vi "Move XYZ.vi"(0 "PID Gains In":T1={"X PID"={"proportional gain (Kc)"=0.03, "integral time (Ti, min)"=0.0, "derivative time (Td, min)"=0.0}, "Y PID"={"proportional gain (Kc)"=0.03, "integral time (Ti, min)"=0.0, "derivative time (Td, min)"=0.0}, "Z PID"={"proportional gain (Kc)"=0.035, "integral time (Ti, min)"=0.0, "derivative time (Td, min)"=0.0}} {"Z PID"."derivative time (Td, min)" format="%.3f"; "Z PID"."integral time (Ti, min)" format="%.3f"; "Z PID"."proportional gain (Kc)" format="%.3f"; "Y PID"."derivative time (Td, min)" format="%.3f"; "Y PID"."integral time (Ti, min)" format="%.3f"; "Y PID"."proportional gain (Kc)" format="%.3f"; "X PID"."derivative time (Td, min)" format="%.3f"; "X PID"."integral time (Ti, min)" format="%.3f"; "X PID"."proportional gain (Kc)" format="%.3f"}, 5 "Y Target":dbl, 6 "X Target":dbl, 10 "Max Time":dbl=90.0, 11 "Gyro Target":dbl=-180.0, 12 "Movement":dbl=3.0, 14 "X Output Range":cluster{"output high":dbl, "output low":dbl}={"output high"=0.8, "output low"=-0.8}, 15 "X Stop Threshold":dbl=5.0, 16 "Y Output Range":cluster{"output high":dbl, "output low":dbl}={"output high"=0.8, "output low"=-0.8}, 17 "Y Stop Threshold":dbl=5.0, 18 "Z Output Range":cluster{"output high":dbl, "output low":dbl}={"output high"=0.8, "output low"=-0.8}, 19 "Z  Stop Threshold":dbl=8.0) -> ()   [LabVIEW 2018]
uses:
  Robot Global Data.vi
  SubSystems/Drive Train/Drive Train Global.vi
  SubSystems/Hatch Panel Intake/Hatch Panel Intake Global.vi
  SubSystems/Lift/Lift Global.vi
  <vilib>/addons/control/pid/pid.llb/PID (DBL).vi
  <vilib>/addons/control/pid/NI_PID_pid.lvlib
panel:
  in  "Minimum Time":u32=500
  in  "Settle Time":u32=2000
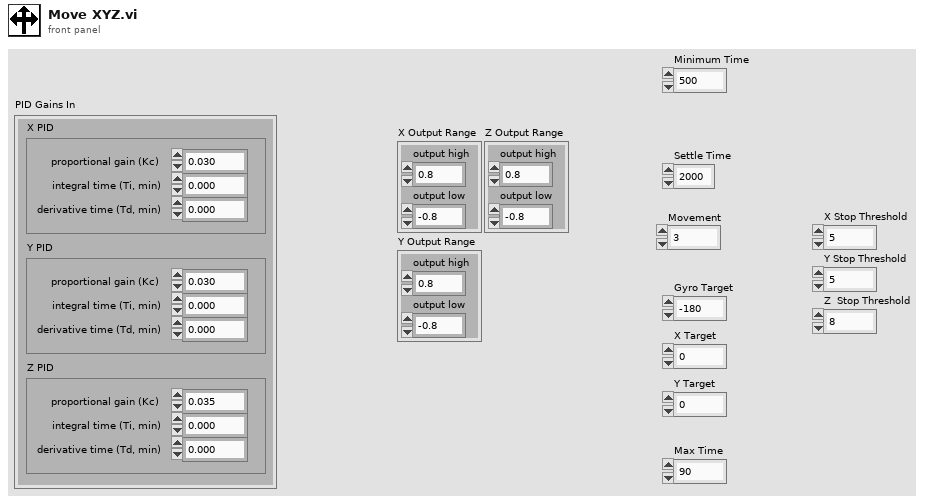
[diagram p1: front panel]
types:
  T1 = cluster{"X PID":cluster{"proportional gain (Kc)":dbl, "integral time (Ti, min)":dbl, "derivative time (Td, min)":dbl}, "Y PID":cluster{"proportional gain (Kc)":dbl, "integral time (Ti, min)":dbl, "derivative time (Td, min)":dbl}, "Z PID":cluster{"proportional gain (Kc)":dbl, "integral time (Ti, min)":dbl, "derivative time (Td, min)":dbl}}
  T2 = cluster{"proportional gain (Kc)":dbl, "integral time (Ti, min)":dbl, "derivative time (Td, min)":dbl}
  T3 = cluster{"Rollover":dbl, "Yaw":dbl, "Cont Yaw":dbl}
  T4 = cluster{"offsetAngle H":dbl, "offsetAngle V":dbl, "area":dbl, "skew":dbl, "validTarget":dbl, "latency":dbl}
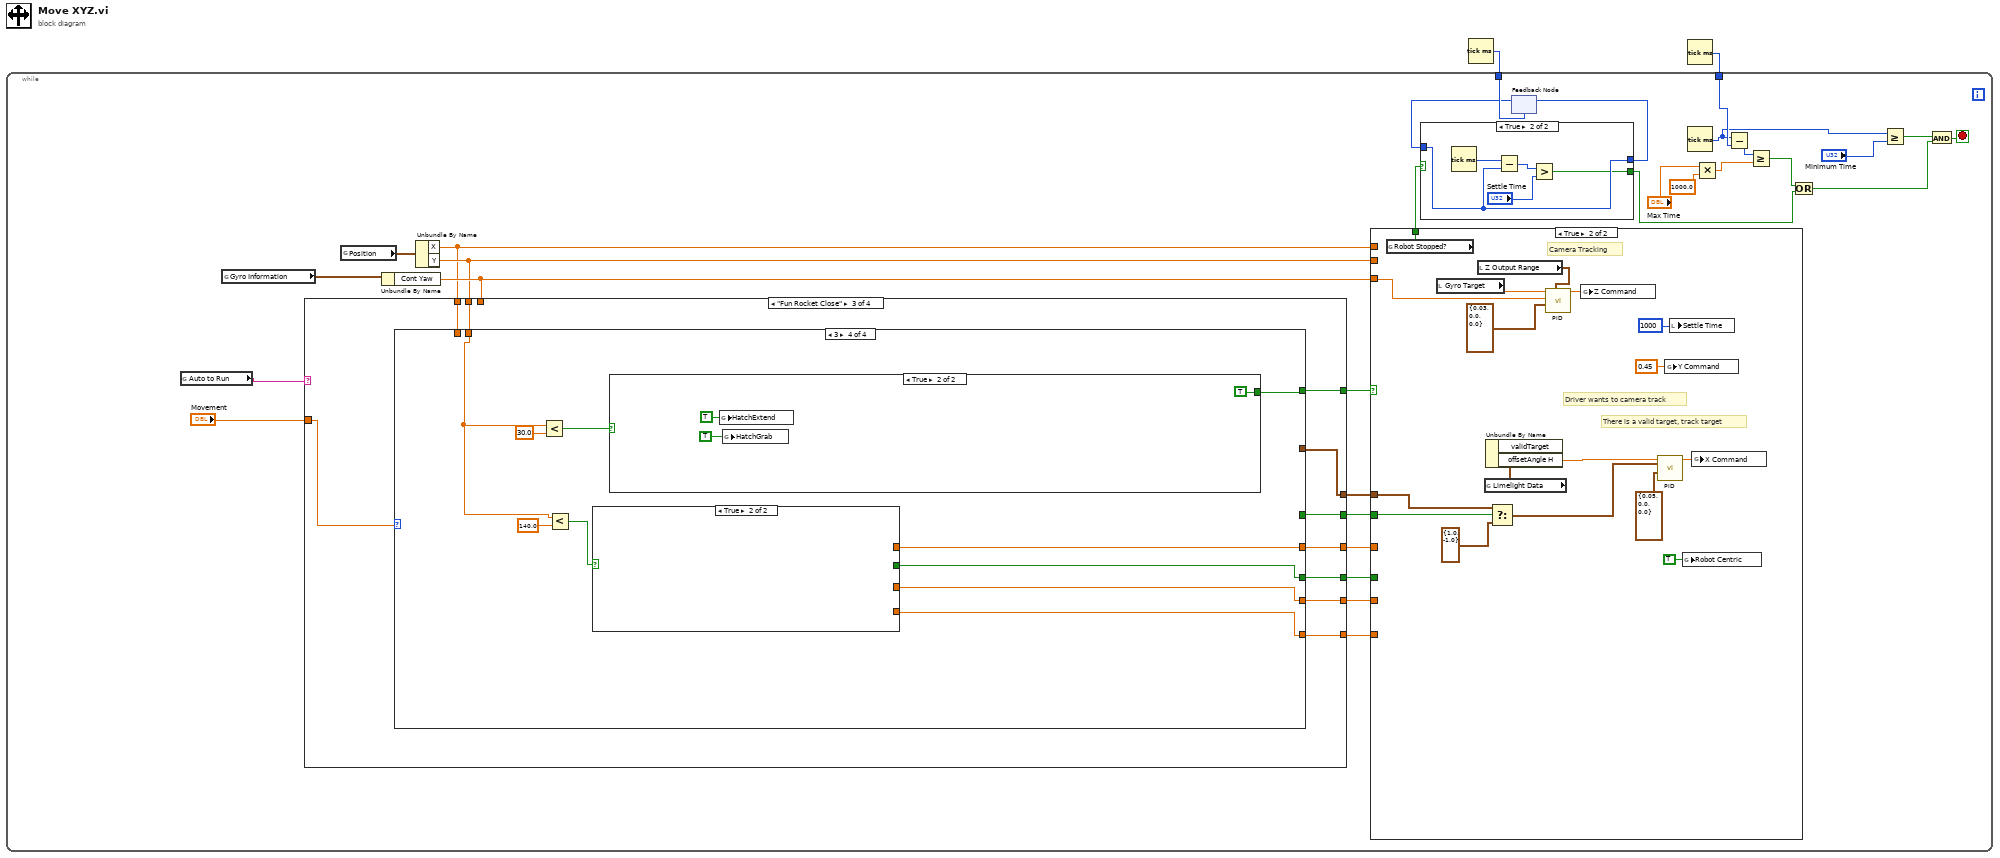
[diagram p0: block diagram]
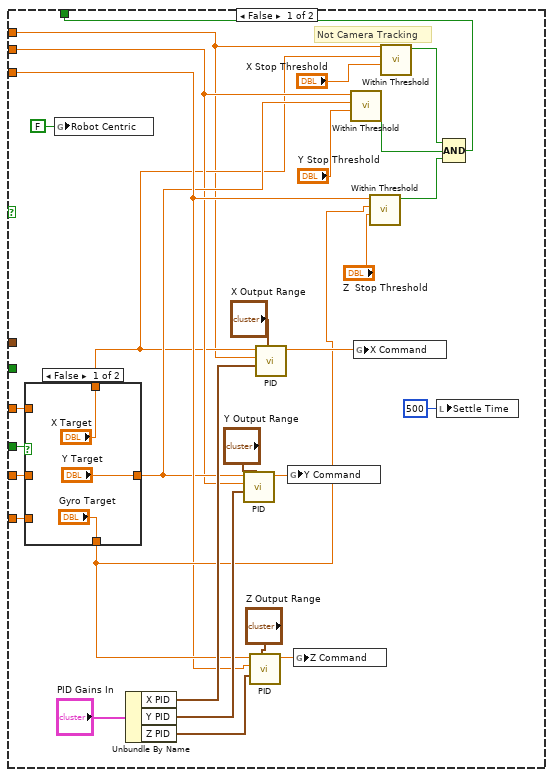
[diagram p2: hidden frame]
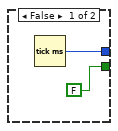
[diagram p4: hidden frame]
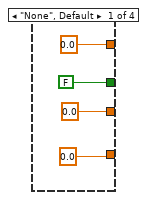
[diagram p5: hidden frame]
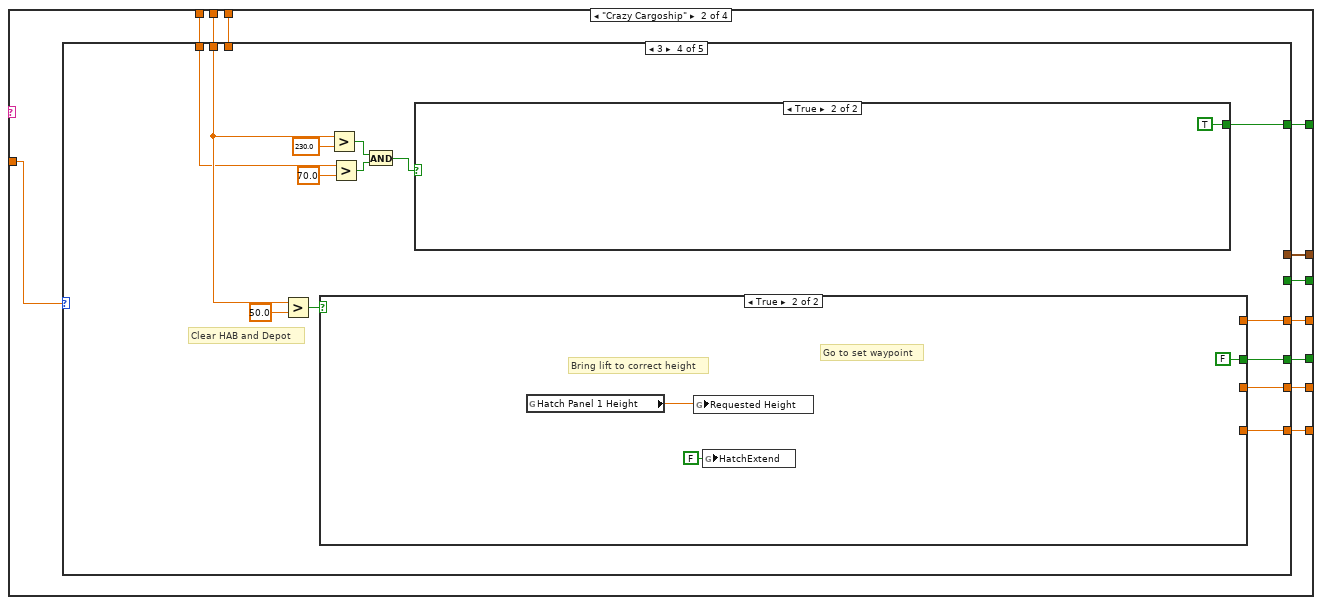
[diagram p6: hidden frame]
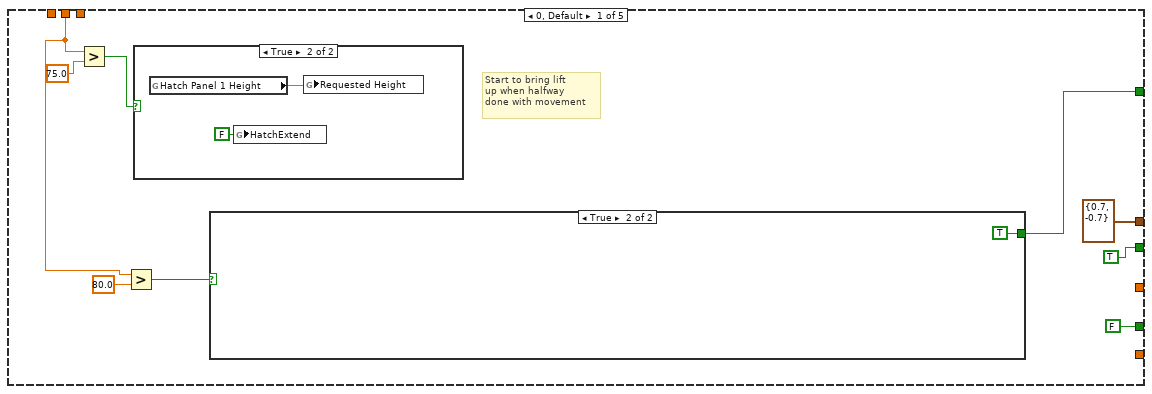
[diagram p7: hidden frame]
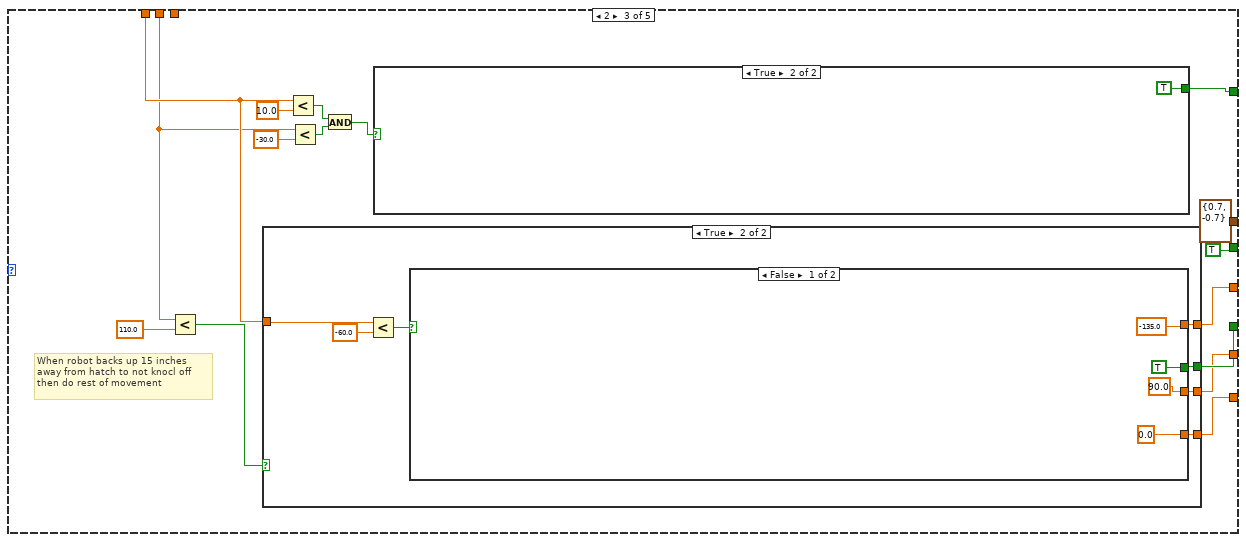
[diagram p11: hidden frame]
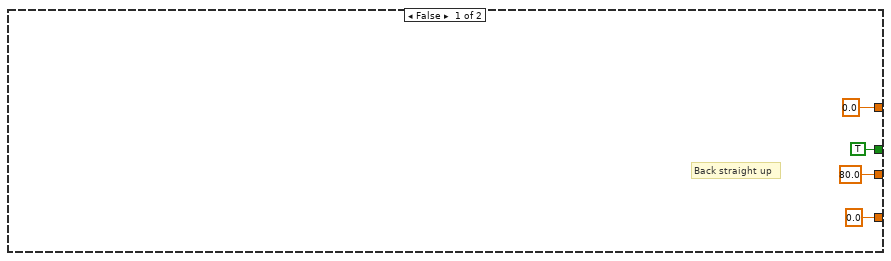
[diagram p13: hidden frame]
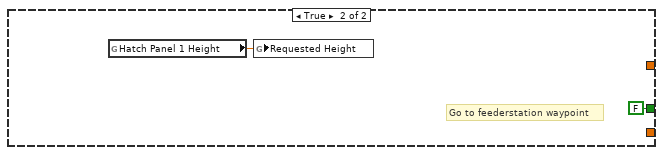
[diagram p14: hidden frame]
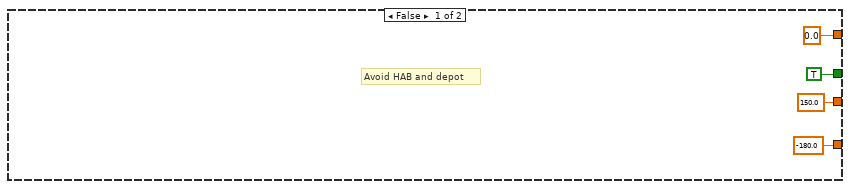
[diagram p16: hidden frame]
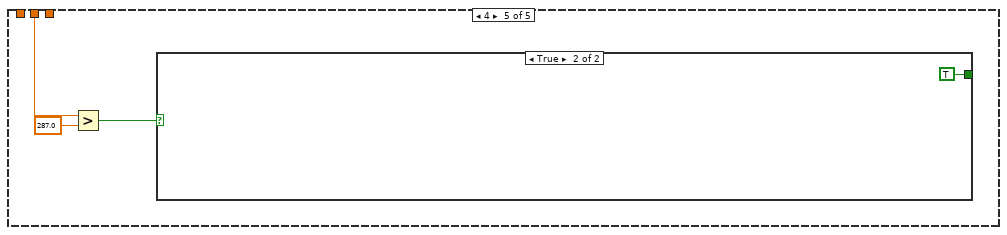
[diagram p17: hidden frame]
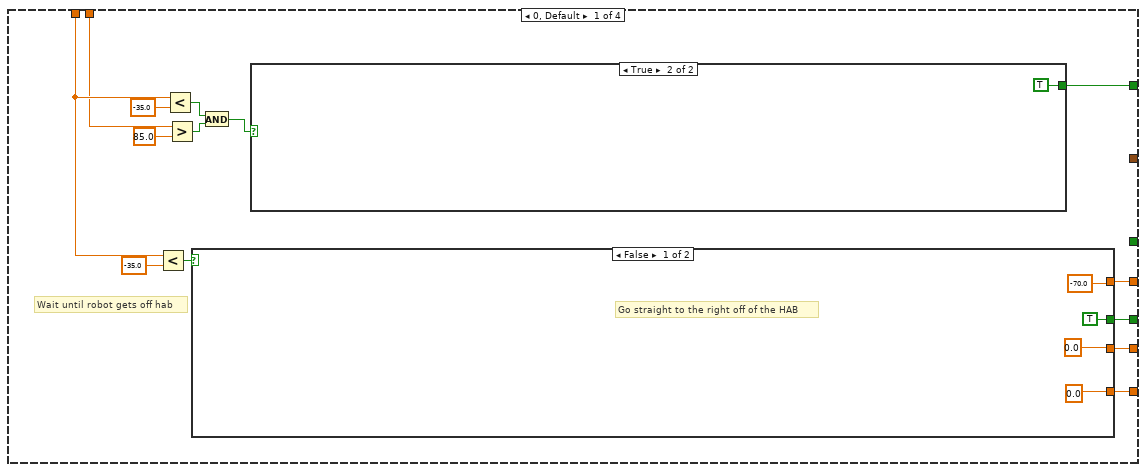
[diagram p19: hidden frame]
diagram:
  n1 = Tick Count (ms)() -> (millisecond timer value=w2:u32)
  n2 = Tick Count (ms)() -> (millisecond timer value=w1:u32)
  n3 = while {
    tunnel: w2 -> [w26]
    tunnel: w1 -> [w11]
    stop <- w10 stop-if-true
    n4 = global read "Robot Global Data.vi" "Auto to Run"() -> (w23:string)
    n5 = global read "Drive Train Global.vi" "Gyro Information"() -> (w20:T3)
    n6 = global read "Drive Train Global.vi" "Position"() -> (w22:cluster{"X":dbl, "Y":dbl})
    n7 = Unbundle By Name(w20) -> ("Cont Yaw"=w18:dbl)
    n8 = Unbundle By Name(w22) -> ("X"=w16:dbl, "Y"=w17:dbl)
    n9 = case shown="\"Fun Rocket Close\"" w23 {
      tunnel: [0.0 w101 w184 w266] -> w32
      tunnel: [0.0 w100 w183 w265] -> w31
      tunnel: [0.0 w99 w182 w264] -> w30
      tunnel: w17 -> [_ w105 w187 w269]
      tunnel: [FALSE w104 w185 w267] -> w29
      tunnel: w16 -> [_ w102 w186 w268]
      tunnel: "Movement" -> [_ w106 w188 w270]
      tunnel: w18 -> [_ w103 _ w262]
      tunnel: [_ w98 w181 w263] -> w5
      tunnel: [_ w96 w179 _] -> w4
      tunnel: [_ w97 w180 _] -> w3
      frame "None", Default {
      }
      frame "Crazy Cargoship" {
        n10 = case shown="3" w106 {
          tunnel: w105 -> [w109 _ w121 w154 w175]
          tunnel: [FALSE _ w132 w166 _] -> w104
          tunnel: w103 -> [_ _ _ _ _]
          tunnel: w102 -> [_ _ w122 w153 _]
          tunnel: [_ _ w131 w163 _] -> w101
          tunnel: [_ _ w130 w162 _] -> w100
          tunnel: [_ _ w129 w161 _] -> w99
          tunnel: [w111 _ w123 w155 _] -> w98
          tunnel: [TRUE ("Robot Centric") _ TRUE ("Robot Centric") _ _] -> w97
          tunnel: [cluster{"output high":dbl, "output low":dbl} {"output high"=0.7, "output low"=-0.7} ("output range") _ cluster{"output high":dbl, "output low":dbl} {"output high"=0.7, "output low"=-0.7} ("output range") _ _] -> w96
          frame 0, Default {
            # "Start to bring lift\nup when halfway\ndone with movement"
            n11 = Greater?(x=w109, y=75.0) -> (0:w114:bool)
            n12 = Greater?(x=w109, y=80.0) -> (0:w110:bool)
            n13 = case shown="True" w114 {
              frame False {
              }
              frame True {
                n14 = global read "Lift Global.vi" "Hatch Panel 1 Height"() -> (w118:dbl)
                n15 = global write "Hatch Panel Intake Global.vi" "HatchExtend"(FALSE ("HatchGrab")) -> ()
                n16 = global write "Lift Global.vi" "Requested Height"(w118) -> ()
              }
            }
            n17 = case shown="True" w110 {
              tunnel: [_ TRUE] -> w111
              frame False {
              }
              frame True {
              }
            }
          }
          frame 1 {
          }
          frame 2 {
            # "When robot backs up 15 inches\naway from hatch to not knocl off\nthen do rest of movement"
            n18 = Less?(x=w121, y=110.0) -> (x < y?=w134:bool)
            n19 = case shown="True" w134 {
              tunnel: [TRUE w146] -> w132
              tunnel: [0.0 w142] -> w131
              tunnel: [80.0 w141] -> w130
              tunnel: [0.0 w140] -> w129
              tunnel: w122 -> [_ w143]
              frame False {
                # "Back straight up"
              }
              frame True {
                n20 = Less?(x=w143, y=-60.0) -> (x < y?=w144:bool)
                n21 = case shown="False" w144 {
                  tunnel: [TRUE FALSE] -> w146
                  tunnel: [-135.0 _] -> w142
                  tunnel: [90.0 _] -> w141
                  tunnel: [0.0 _] -> w140
                  frame False {
                  }
                  frame True {
                    # "Go to feederstation waypoint"
                    n22 = global read "Lift Global.vi" "Hatch Panel 1 Height"() -> (w151:dbl)
                    n23 = global write "Lift Global.vi" "Requested Height"(w151) -> ()
                  }
                }
              }
            }
            n24 = Less?(x=w122, y=10.0) -> (x < y?=w126:bool)
            n25 = Less?(x=w121, y=-30.0) -> (x < y?=w125:bool)
            n26 = And(x=w126, y=w125) -> (x .and. y?=w124:bool)
            n27 = case shown="True" w124 {
              tunnel: [_ TRUE] -> w123
              frame False {
              }
              frame True {
              }
            }
          }
          frame 3 {
            # "Clear HAB and Depot"
            n28 = Greater?(x=w154, y=50.0) -> (0:w165:bool)
            n29 = case shown="True" w165 {
              tunnel: [TRUE FALSE] -> w166
              tunnel: [0.0 _] -> w163
              tunnel: [150.0 _] -> w162
              tunnel: [-180.0 _] -> w161
              frame False {
                # "Avoid HAB and depot"
              }
              frame True {
                # "Bring lift to correct height"
                # "Go to set waypoint"
                n30 = global read "Lift Global.vi" "Hatch Panel 1 Height"() -> (w173:dbl)
                n31 = global write "Lift Global.vi" "Requested Height"(w173) -> ()
                n32 = global write "Hatch Panel Intake Global.vi" "HatchExtend"(FALSE ("HatchGrab")) -> ()
              }
            }
            n33 = Greater?(x=w154, y=230.0) -> (0:w158:bool)
            n34 = Greater?(x=w153, y=70.0) -> (0:w157:bool)
            n35 = And(x=w158, y=w157) -> (x .and. y?=w156:bool)
            n36 = case shown="True" w156 {
              tunnel: [_ TRUE] -> w155
              frame False {
              }
              frame True {
              }
            }
          }
          frame 4 {
            n37 = Greater?(x=w175, y=287.0) -> (0:w176:bool)
            n38 = case shown="True" w176 {
              tunnel: [_ TRUE] -> _
              frame False {
              }
              frame True {
              }
            }
          }
        }
      }
      frame "Fun Rocket Close" {
        n39 = case shown="3" w188 {
          tunnel: w187 -> [w195 w210 w229 w250]
          tunnel: w186 -> [w196 w215 _ _]
          tunnel: [w200 _ w227 w245] -> w185
          tunnel: [w199 _ w228 w248] -> w184
          tunnel: [w198 _ w226 w247] -> w183
          tunnel: [w197 _ w225 w246] -> w182
          tunnel: [w189 w216 w235 w253] -> w181
          tunnel: [_ _ w233 _] -> w180
          tunnel: [_ _ w232 _] -> w179
          frame 0, Default {
            # "Wait until robot gets off hab"
            n40 = Less?(x=w196, y=-35.0) -> (x < y?=w202:bool)
            n41 = Less?(x=w196, y=-35.0) -> (x < y?=w192:bool)
            n42 = Greater?(x=w195, y=85.0) -> (0:w191:bool)
            n43 = case shown="False" w202 {
              tunnel: [TRUE FALSE] -> w200
              tunnel: [-70.0 _] -> w199
              tunnel: [0.0 _] -> w198
              tunnel: [0.0 _] -> w197
              frame False {
                # "Go straight to the right off of the HAB"
              }
              frame True {
                # "Bring the lift up to the correct level because its slow"
                # "Robot off of HAB, go to the rocket"
                n44 = global read "Lift Global.vi" "Hatch Panel 2 Height"() -> (w208:dbl)
                n45 = global write "Lift Global.vi" "Requested Height"(w208) -> ()
              }
            }
            n46 = And(x=w192, y=w191) -> (x .and. y?=w190:bool)
            n47 = case shown="True" w190 {
              tunnel: [_ TRUE] -> w189
              frame False {
              }
              frame True {
              }
            }
          }
          frame 1 {
            n48 = Less?(x=w210, y=-17.0) -> (x < y?=w219:bool)
            n49 = Less?(x=w215, y=-90.0) -> (x < y?=w218:bool)
            n50 = Less?(x=w210, y=0.0) -> (x < y?=w213:bool)
            n51 = Less?(x=w210, y=-5.0) -> (x < y?=w212:bool)
            n52 = And(x=w219, y=w218) -> (x .and. y?=w217:bool)
            n53 = case shown="True" w213 {
              frame False {
              }
              frame True {
                n54 = global write "Hatch Panel Intake Global.vi" "HatchExtend"(TRUE ("HatchExtend")) -> ()
              }
            }
            n55 = case shown="True" w212 {
              frame False {
              }
              frame True {
                n56 = global write "Hatch Panel Intake Global.vi" "HatchGrab"(TRUE ("HatchExtend")) -> ()
              }
            }
            n57 = case shown="True" w217 {
              tunnel: [_ TRUE] -> w216
              frame False {
              }
              frame True {
              }
            }
          }
          frame 2 {
            # "back up then turn"
            n58 = Greater?(x=w229, y=150.0) -> (0:w234:bool)
            n59 = Greater?(x=w229, y=40.0) -> (0:w230:bool)
            n60 = case shown="True" w234 {
              tunnel: [_ TRUE] -> w235
              tunnel: [_ TRUE] -> w233
              tunnel: [_ cluster{"output high":dbl, "output low":dbl} {"output high"=0.6, "output low"=-0.6} ("output range")] -> w232
              frame False {
              }
              frame True {
              }
            }
            n61 = case shown="False" w230 {
              tunnel: [0.0 _] -> w228
              tunnel: [TRUE FALSE] -> w227
              tunnel: [200.0 _] -> w226
              tunnel: [-180.0 _] -> w225
              frame False {
              }
              frame True {
              }
            }
          }
          frame 3 {
            n62 = Less?(x=w250, y=30.0) -> (x < y?=w252:bool)
            n63 = Less?(x=w250, y=140.0) -> (x < y?=w249:bool)
            n64 = case shown="True" w249 {
              tunnel: [0.0 _] -> w248
              tunnel: [100.0 _] -> w247
              tunnel: [-30.0 _] -> w246
              tunnel: [TRUE _] -> w245
              frame False {
              }
              frame True {
              }
            }
            n65 = case shown="True" w252 {
              tunnel: [_ TRUE] -> w253
              frame False {
              }
              frame True {
                n66 = global write "Hatch Panel Intake Global.vi" "HatchExtend"(TRUE ("HatchExtend")) -> ()
                n67 = global write "Hatch Panel Intake Global.vi" "HatchGrab"(TRUE ("HatchExtend")) -> ()
              }
            }
          }
        }
      }
      frame "Fun Rocket Far" {
        n68 = case shown="2" w270 {
          tunnel: w269 -> [w273 w307 w326 w342]
          tunnel: w268 -> [w272 w305 _ _]
          tunnel: [w277 w303 w331 w337] -> w267
          tunnel: [w276 w304 w330 w340] -> w266
          tunnel: [w275 w302 w329 w339] -> w265
          tunnel: [w274 w301 w328 w338] -> w264
          tunnel: [w271 w310 _ w345] -> w263
          tunnel: w262 -> [_ _ _ _]
          frame 0, Default {
            # "Wait until robot gets off hab"
            n69 = Greater?(x=w273, y=160.0) -> (0:w279:bool)
            n70 = case shown="True" w279 {
              tunnel: [TRUE w292] -> w277
              tunnel: [-10.0 w290] -> w276
              tunnel: [170.0 w289] -> w275
              tunnel: [0.0 w288] -> w274
              tunnel: w272 -> [_ w285]
              tunnel: [_ w284] -> w271
              frame False {
              }
              frame True {
                # "Bring the lift up to the correct level because its slow"
                n71 = global read "Lift Global.vi" "Hatch Panel 2 Height"() -> (w291:dbl)
                n72 = global write "Lift Global.vi" "Requested Height"(w291) -> ()
                n73 = Less?(x=w285, y=-60.0) -> (x < y?=w286:bool)
                n74 = case shown="False" w286 {
                  tunnel: [TRUE FALSE] -> w292
                  tunnel: [-100.0 ("y") _] -> w290
                  tunnel: [195.0 ("y") _] -> w289
                  tunnel: [-150.0 ("y") _] -> w288
                  tunnel: [_ TRUE] -> w284
                  frame False {
                  }
                  frame True {
                  }
                }
              }
            }
          }
          frame 1 {
            n75 = Less?(x=w307, y=-30.0) -> (x < y?=w313:bool)
            n76 = Greater?(x=w305, y=65.0) -> (0:w312:bool)
            n77 = Less?(x=w307, y=0.0) -> (x < y?=w308:bool)
            n78 = And(x=w313, y=w312) -> (x .and. y?=w311:bool)
            n79 = case shown="True" w308 {
              frame False {
              }
              frame True {
                n80 = global write "Hatch Panel Intake Global.vi" "HatchExtend"(TRUE ("HatchExtend")) -> ()
                n81 = global write "Hatch Panel Intake Global.vi" "HatchGrab"(TRUE ("HatchExtend")) -> ()
              }
            }
            n82 = Greater?(x=w305, y=-40.0) -> (0:w299:bool)
            n83 = case shown="False" w311 {
              tunnel: [FALSE TRUE] -> w310
              frame False {
              }
              frame True {
              }
            }
            n84 = call "Flip Flop.vi"("Line 1"=w299) -> ("Switch"=w300:bool)  [unwired: 10 in]
            n85 = case shown="True" w300 {
              tunnel: [_ -30.0 ("y")] -> w304
              tunnel: [FALSE TRUE] -> w303
              tunnel: [_ 190.0 ("y")] -> w302
              tunnel: [_ -150.0 ("y")] -> w301
              frame False {
              }
              frame True {
              }
            }
          }
          frame 2 {
            n86 = Less?(x=w326, y=30.0) -> (x < y?=w327:bool)
            n87 = case shown="False" w327 {
              tunnel: [TRUE FALSE] -> w331
              tunnel: [-30.0 _] -> w330
              tunnel: [100.0 _] -> w329
              tunnel: [-180.0 _] -> w328
              frame False {
              }
              frame True {
              }
            }
          }
          frame 3 {
            n88 = Less?(x=w342, y=30.0) -> (x < y?=w344:bool)
            n89 = Less?(x=w342, y=140.0) -> (x < y?=w341:bool)
            n90 = case shown="False" w341 {
              tunnel: [0.0 _] -> w340
              tunnel: [100.0 _] -> w339
              tunnel: [-30.0 _] -> w338
              tunnel: [TRUE _] -> w337
              frame False {
              }
              frame True {
              }
            }
            n91 = case shown="True" w344 {
              tunnel: [_ TRUE] -> w345
              frame False {
              }
              frame True {
              }
            }
          }
        }
      }
    }
    n92 = case shown="True" w5 {
      tunnel: w32 -> [w54 _]
      tunnel: w31 -> [w53 _]
      tunnel: w30 -> [w52 _]
      tunnel: w29 -> [w51 _]
      tunnel: [w35 w68] -> w19
      tunnel: w18 -> [w45 w75]
      tunnel: w17 -> [w41 _]
      tunnel: w16 -> [w37 _]
      tunnel: w4 -> [_ w71]
      tunnel: w3 -> [_ w70]
      frame False {
        # "Not Camera Tracking"
        n93 = case shown="False" w51 {
          tunnel: ["X Target" w67] -> w38
          tunnel: ["Y Target" w66] -> w42
          tunnel: ["Gyro Target" w65] -> w46
          tunnel: w54 -> [_ w67]
          tunnel: w53 -> [_ w66]
          tunnel: w52 -> [_ w65]
          frame False {
          }
          frame True {
          }
        }
        n94 = global write "Drive Train Global.vi" "Robot Centric"(FALSE ("Robot Centric")) -> ()
        n95 = Unbundle By Name("PID Gains In") -> ("X PID"=w59:T2, "Y PID"=w58:T2, "Z PID"=w57:T2)
        n96 = call-poly <vilib>:"PID.vi"("output range"="Y Output Range", "PID gains"=w58, "process variable"=w41, "setpoint"=w42) -> ("output"=w48:dbl)  [unwired: 6 in, 1 out]
        n97 = call-poly <vilib>:"PID.vi"("output range"="Z Output Range", "PID gains"=w57, "process variable"=w45, "setpoint"=w46) -> ("output"=w49:dbl)  [unwired: 6 in, 1 out]
        n98 = call-poly <vilib>:"PID.vi"("output range"="X Output Range", "PID gains"=w59, "process variable"=w37, "setpoint"=w38) -> ("output"=w50:dbl)  [unwired: 6 in, 1 out]
        n99 = global write "Drive Train Global.vi" "Y Command"(w48) -> ()
        n100 = global write "Drive Train Global.vi" "Z Command"(w49) -> ()
        n101 = call "Within Threshold.vi"("Threshold"="Y Stop Threshold", "Center"=w42, "Value"=w41) -> ("Within Threshold?"=w43:bool)  [unwired: 8 in]
        n102 = global write "Drive Train Global.vi" "X Command"(w50) -> ()
        n103 = call "Within Threshold.vi"("Threshold"="Z  Stop Threshold", "Center"=w46, "Value"=w45) -> ("Within Threshold?"=w47:bool)  [unwired: 8 in]
        n104 = call "Within Threshold.vi"("Threshold"="X Stop Threshold", "Center"=w38, "Value"=w37) -> ("Within Threshold?"=w39:bool)  [unwired: 8 in]
        n105 = local write "Settle Time"(u32 500 ("Settle Time")) -> ()
        n106 = Compound Arithmetic op=AND(w39, w43, w47) -> (w35:bool)
      }
      frame True {
        # "There is a valid target, track target"
        # "Driver wants to camera track"
        # "Camera Tracking"
        n107 = global read "Drive Train Global.vi" "Robot Stopped?"() -> (w68:bool)
        n108 = local read "Gyro Target"() -> (w76:dbl)
        n109 = local read "Z Output Range"() -> (w77:cluster{"output high":dbl, "output low":dbl})
        n110 = global read "Robot Global Data.vi" "Limelight Data"() -> (w82:T4)
        n111 = Unbundle By Name(w82) -> ("offsetAngle H"=w81:dbl)  [unwired: 1 out]
        n112 = Select(t=w71, s=w70, f=cluster{"output high":dbl, "output low":dbl} {"output high"=1.0, "output low"=-1.0} ("output range")) -> (s? t:f=w72:cluster{"output high":dbl, "output low":dbl})
        n113 = call-poly <vilib>:"PID.vi"("output range"=w77, "PID gains"=T2 {"proportional gain (Kc)"=0.03, "integral time (Ti, min)"=0.0, "derivative time (Td, min)"=0.0}, "process variable"=w75, "setpoint"=w76) -> ("output"=w78:dbl)  [unwired: 6 in, 1 out]
        n114 = global write "Drive Train Global.vi" "Z Command"(w78) -> ()
        n115 = call-poly <vilib>:"PID.vi"("output range"=w72, "PID gains"=T2 {"proportional gain (Kc)"=0.05, "integral time (Ti, min)"=0.0, "derivative time (Td, min)"=0.0} ("Camera Tracking"), "setpoint"=w81) -> ("output"=w83:dbl)  [unwired: 7 in, 1 out]
        n116 = global write "Drive Train Global.vi" "Y Command"(0.45 ("Y Command")) -> ()
        n117 = local write "Settle Time"(u32 1000 ("Settle Time")) -> ()
        n118 = global write "Drive Train Global.vi" "Robot Centric"(TRUE ("Robot Centric")) -> ()
        n119 = global write "Drive Train Global.vi" "X Command"(w83) -> ()
      }
    }
    n120 = feedback #1(w26) -> (w25:u32)
    n121 = case shown="True" w19 {
      tunnel: [w86 w89] -> w27
      tunnel: w25 -> [_ w89]
      tunnel: [FALSE w88] -> w24
      frame False {
        n122 = Tick Count (ms)() -> (millisecond timer value=w86:u32)
      }
      frame True {
        n123 = Tick Count (ms)() -> (millisecond timer value=w91:u32)
        n124 = Subtract(x=w91, y=w89) -> (x-y=w90:u32)
        n125 = Greater?(x=w90, y="Settle Time") -> (0:w88:bool)
      }
    }
    n126 = feedback-in #1(w27) -> ()
    n127 = Tick Count (ms)() -> (millisecond timer value=w9:u32)
    n128 = Multiply(x="Max Time", y=1000.0) -> (x*y=w14:dbl)
    n129 = Subtract(x=w9, y=w11) -> (x-y=w15:u32)
    n130 = Greater Or Equal?(x=w15, y=w14) -> (x >= y?=w28:bool)
    n131 = Or(x=w28, y=w24) -> (x .or. y?=w6:bool)
    n132 = Greater Or Equal?(x=w9, y="Minimum Time") -> (x >= y?=w7:bool)
    n133 = And(x=w7, y=w6) -> (x .and. y?=w10:bool)
  }
